vi "getCost.vi"(8 "error in (no error)":errorcluster, 11 "Decaf in":refnum<class "Decaf.lvclass">) -> (0 "error out":errorcluster, 2 "cost":dbl, 3 "Decaf out":refnum<class "Decaf.lvclass">)   [LabVIEW 2017, in "Decaf.lvclass"]
uses:
  Decaf.lvclass
  Beverage Class/Beverage.lvclass
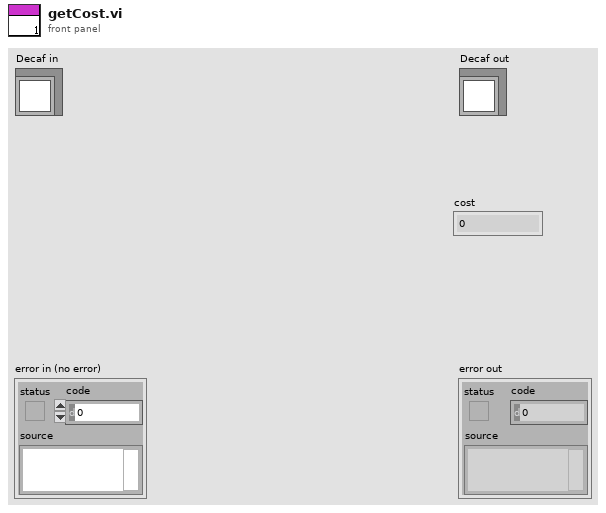
[diagram p1: front panel]
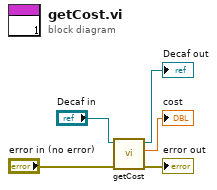
[diagram p0: block diagram]
diagram:
  n1 = call-parent "getCost.vi"("error in (no error)"="error in (no error)", "Beverage in"="Decaf in") -> ("error out"=→"error out":errorcluster, "cost"=→"cost":dbl, "Beverage out"=→"Decaf out":refnum<class "Decaf.lvclass">)  [unwired: 7 in]
